vi "LWXPS_GroupPositionCurrentGet.vi"(0 "XPS Reference IN":refnum<k24>, 5 "Group Name":string, 7 "Number of positioners":i32, 11 "LabVIEW error IN":errorcluster) -> (4 "XPS Reference OUT":refnum<k24>, 6 "Returned error code":i32, 8 "Current Encoder Position":dbl[](array[numeric]), 10 "XPS Error String":string, 15 "LabVIEW error OUT":errorcluster)   [LabVIEW 2020]
uses:
  C:/GEECS/Developers Version/source/Device Drivers/NewportXPS/XPS-RLD/XPS-UNIFIED/LabVIEW VIs/LabVIEW Source Code/Dll/Newport.XPS.CommandInterface.dll
  Dll/Newport.XPS.CommandInterface.dll
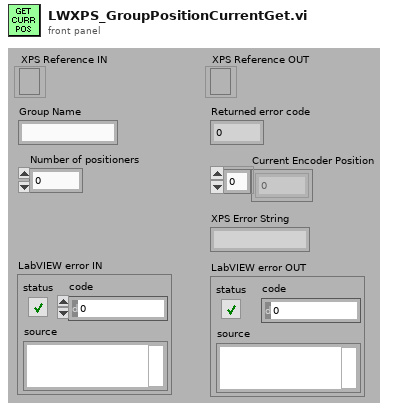
[diagram p1: front panel]
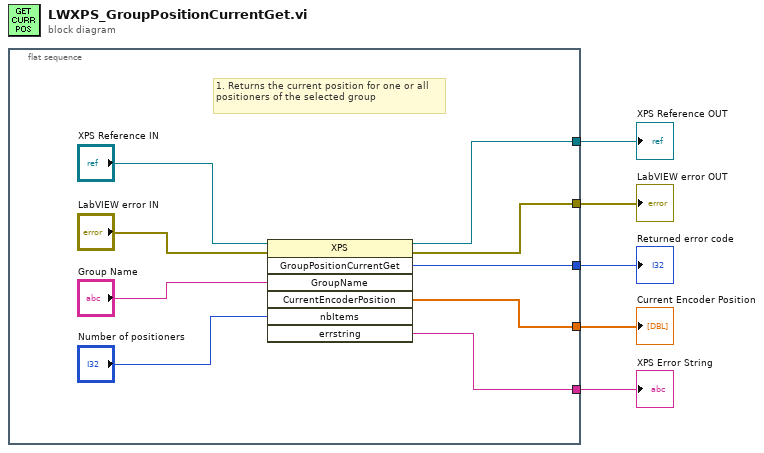
[diagram p0: block diagram]
diagram:
  n1 = flat-sequence {
    tunnel: [w9] -> w5
    tunnel: [w11] -> w4
    tunnel: [w13] -> w3
    tunnel: [w7] -> w2
    tunnel: [w8] -> w1
    frame #0 {
      # "1. Returns the current position for one or all positioners of the selected group"
      n2 = invoke class="XPS" method="GroupPositionCurrentGet"(reference="XPS Reference IN", error in="LabVIEW error IN", "GroupName"="Group Name", "nbItems"="Number of positioners") -> (reference out=w9:refnum<k24>, error out=w11:errorcluster, "GroupPositionCurrentGet"=w13:i32, "CurrentEncoderPosition"=w8:dbl[], "errstring"=w7:string)  [unwired: 3 in, 2 out]
    }
  }
  "XPS Reference OUT" <- w5
  "LabVIEW error OUT" <- w4
  "Returned error code" <- w3
  "XPS Error String" <- w2
  "Current Encoder Position" <- w1
